vi "Constructor.vi"(8 "error in (no error)":errorcluster, 11 "device index":i32) -> (0 "error out":errorcluster, 2 "Joystick":refnum<event-registration>, 3 "Mouse out":refnum<class "Joystick.lvclass">)   [LabVIEW 2021, in "InputDevice.lvlib" / "Joystick.lvclass"]
uses:
  Joystick.lvclass
  Joystick.lvclass/Joystick.ctl
  data.ctl
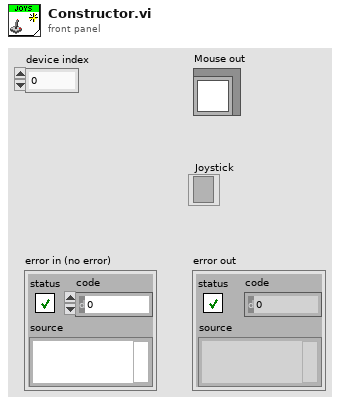
[diagram p1: front panel]
types:
  T1 = typedef "InputDevice.lvlib/Joystick.lvclass/data.ctl" = cluster{"DeviceID":refnum<k1>, "JoyButtonInfo":refnum<user-event>, "JoyAxisInfo":refnum<user-event>, "JoyDirectionInfo":refnum<user-event>, "Joystick":refnum<event-registration>, "StopNotifier":refnum<notifier>}
  T2 = cluster{"X axis":i32, "Y axis":i32, "Z axis":i32, "X axis rotation":i32, "Y axis rotation":i32, "Z axis rotation":i32, "U axis":i32, "V axis":i32}
  T3 = cluster{"pov 1":i32, "pov 2":i32, "pov 3":i32, "pov 4":i32}
  T4 = cluster{"button 1":bool, "button 2":bool, "button 3":bool, "button 4":bool, "button 5":bool, "button 6":bool, "button 7":bool, "button 8":bool, "button 9":bool, "button 10":bool, "button 11":bool, "button 12":bool, "button 13":bool, "button 14":bool, "button 15":bool, "button 16":bool, "button 17":bool, "button 18":bool, "button 19":bool, "button 20":bool, "button 21":bool, "button 22":bool, "button 23":bool, "button 24":bool, "button 25":bool, "button 26":bool, "button 27":bool, "button 28":bool, "button 29":bool, "button 30":bool, "button 31":bool, "button 32":bool}
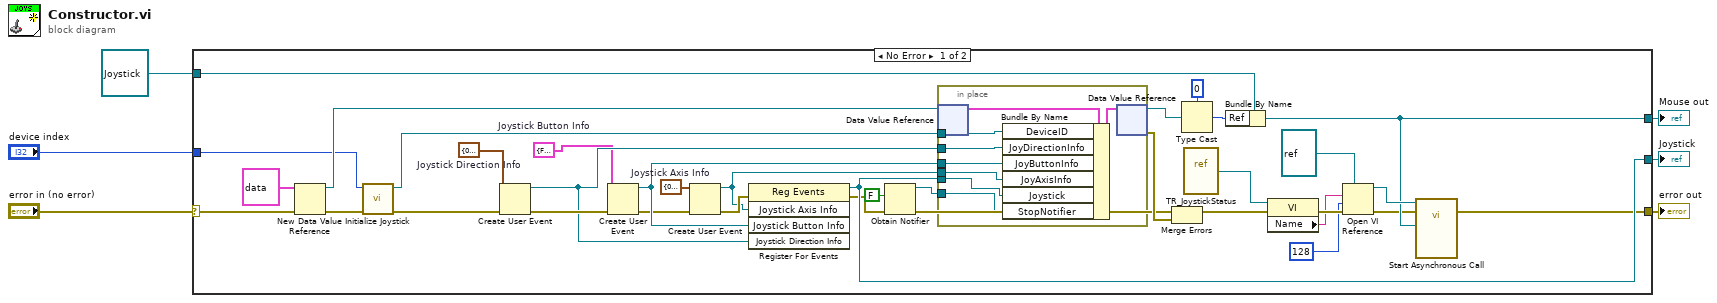
[diagram p0: block diagram]
diagram:
  n1 = case shown="No Error" "error in (no error)" {
    selector: "error in (no error)" -> [w36 w52]
    tunnel: [w15 w52] -> w5
    tunnel: [w17 w51] -> w4
    tunnel: refnum<class "Joystick.lvclass"> refnum ("Joystick.lvclass") -> [w40 w51]
    tunnel: [w28 _] -> w2
    tunnel: "device index" -> [w7 _]
    frame No Error {
      w9 = T2 {"X axis"=0, "Y axis"=0, "Z axis"=0, "X axis rotation"=0, "Y axis rotation"=0, "Z axis rotation"=0, "U axis"=0, "V axis"=0}  # Joystick Axis Info
      w12 = T3 {"pov 1"=0, "pov 2"=0, "pov 3"=0, "pov 4"=0}  # Joystick Direction Info
      w13 = T4 {"button 1"=FALSE, "button 2"=FALSE, "button 3"=FALSE, "button 4"=FALSE, "button 5"=FALSE, "button 6"=FALSE, "button 7"=FALSE, "button 8"=FALSE, "button 9"=FALSE, "button 10"=FALSE, "button 11"=FALSE, "button 12"=FALSE, "button 13"=FALSE, "button 14"=FALSE, "button 15"=FALSE, "button 16"=FALSE, "button 17"=FALSE, "button 18"=FALSE, "button 19"=FALSE, "button 20"=FALSE, "button 21"=FALSE, "button 22"=FALSE, "button 23"=FALSE, "button 24"=FALSE, "button 25"=FALSE, "button 26"=FALSE, "button 27"=FALSE, "button 28"=FALSE, "button 29"=FALSE, "button 30"=FALSE, "button 31"=FALSE, "button 32"=FALSE}  # Joystick Button Info
      n2 = New Data Value Reference(data value=T1 {"DeviceID"=refnum, "JoyButtonInfo"=refnum, "JoyAxisInfo"=refnum, "JoyDirectionInfo"=refnum, "Joystick"=refnum, "StopNotifier"=refnum} ("Cluster"), error in=w36) -> (data value reference=w41:refnum<data-value>, error out=w35:errorcluster)
      n3 = call <vilib>:"Initialize Joystick.vi"("error in (no error)"=w35, "device index"=w7) -> ("error out"=w32:errorcluster, "device ID"=w34:refnum<k1>)  [unwired: 8 in]
      n4 = Create User Event(user event datatype=w12, error in=w32) -> (user event=w29:refnum<user-event>, error out=w31:errorcluster)
      n5 = Create User Event(user event datatype=w13, error in=w31) -> (user event=w30:refnum<user-event>, error out=w11:errorcluster)
      n6 = Create User Event(user event datatype=w9, error in=w11) -> (user event=w8:refnum<user-event>, error out=w10:errorcluster)
      n7 = register-events(error in=w10, w8, w30, w29) -> (reference out=w28:refnum<event-registration>, error out=w26:errorcluster)  [unwired: 1 in]
      n8 = Obtain Notifier(notification data type=FALSE, error in (no error)=w26) -> (notifier out=w14:refnum<notifier>, error out=w25:errorcluster)  [unwired: 2 in, 1 out]
      n9 = in-place {
        in-place-border: w34 -> [w48]
        in-place-border: w29 -> [w47]
        in-place-border: w30 -> [w46]
        in-place-border: w28 -> [w43]
        in-place-border: w14 -> [w45]
        in-place-border: w8 -> [w44]
        n10 = in-place-dvr #1(w41) -> (w50:T1)  [unwired: 1 out]
        n11 = Bundle By Name(cluster=w50, "DeviceID"=w48, "JoyDirectionInfo"=w47, "JoyButtonInfo"=w46, "JoyAxisInfo"=w44, "Joystick"=w43, "StopNotifier"=w45) -> (w49:T1)
        n12 = in-place-dvr #1(w49) -> (w39:refnum<data-value>, w33:errorcluster)
      }
      n13 = Merge Errors(w25, w33) -> (w24:errorcluster)
      n14 = Type Cast(type=u64 0 ("Ref"), x=w39) -> (*(type *) &x=w37:u64)
      n15 = vi-ref "TR_JoystickStatus.vi"() -> (w20:refnum<vi>)
      n16 = Bundle By Name(cluster=w40, "Ref"=w37) -> (w17:refnum<class "Joystick.lvclass">)
      n17 = property class="VI"(reference=w20, error in=w24) -> (error out=w23:errorcluster, "Name"=w22:string)  [unwired: 1 out]
      n18 = Open VI Reference(type specifier VI Refnum (for type only)=refnum<vi> refnum, vi path=w22, options=128, error in (no error)=w23) -> (vi reference=w19:refnum<vi>, error out=w16:errorcluster)  [unwired: 2 in]
      n19 = call-by-ref "Start Asynchronous Call"(reference=w19, error in=w16, "Mouse in"=w17) -> (error out=w15:errorcluster)  [unwired: 11 in, 1 out]
    }
    frame Error {
    }
  }
  "error out" <- w5
  "Mouse out" <- w4
  "Joystick" <- w2
